vi "OAT Multistage Interpolation with IC.vi"(6 "initial state":cluster{"initial state":dbl[]}[](array[cluster]) {"initial state" format="%.2f"}, 8 "error in (no error)":errorcluster, 9 "filter":T1[](array[typedef]) {"coefficients" format="%.2f"}, 11 "X":dbl[](array[numeric]) format="%.2f") -> (0 "error out":errorcluster, 3 "Y":dbl[](array[numeric]) format="%.2f", 4 "final state":cluster{"final state":dbl[]}[](array[cluster]) {"final state" format="%.2f"})   [LabVIEW 2017, in "SoundVib_Resampling.lvlib"]
doc: "Interpolate the input sequence <B>X</B> with the multistage interpolation filter specified by <B>filter</B>."
uses:
  <vilib>/addons/Sound and Vibration/Order Analysis/Resample Order Tracking/SoundVib_Resampling.lvlib
  <vilib>/addons/_NISVFA/_Shared subVIs/Controls/OAT Decimation Filter.ctl
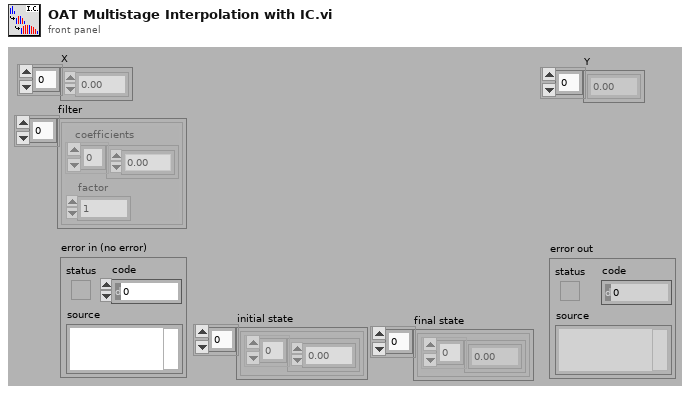
[diagram p1: front panel]
types:
  T1 = typedef "OAT Decimation Filter.ctl" = cluster{"coefficients":dbl[], "factor":i32}
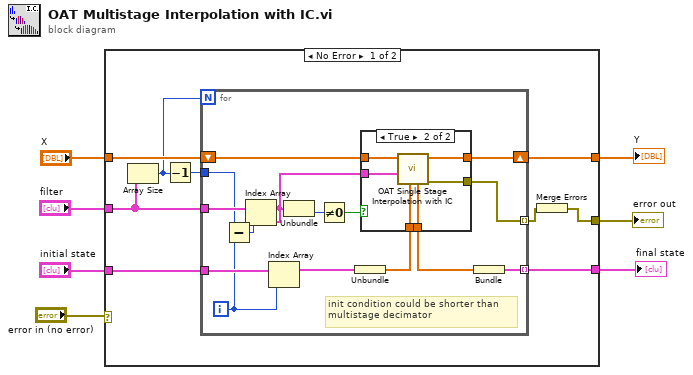
[diagram p0: block diagram]
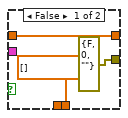
[diagram p2: hidden frame]
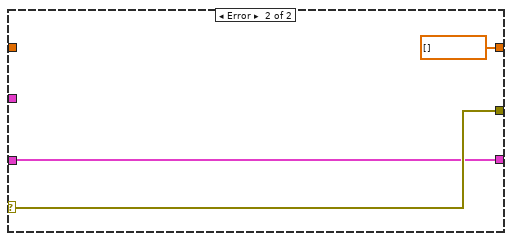
[diagram p3: hidden frame]
diagram:
  n1 = case shown="No Error" "error in (no error)" {
    selector: "error in (no error)" -> [_ w43]
    tunnel: "X" -> [w16 _]
    tunnel: [w15 w41] -> w6
    tunnel: [w14 dbl[] [] ("X")] -> w5
    tunnel: "initial state" -> [w13 w41]
    tunnel: "filter" -> [w12 _]
    tunnel: [w8 w43] -> w2
    frame No Error {
      n2 = Array Size(array=w12) -> (size(s)=w11:i32)
      n3 = Decrement(x=w11) -> (x-1=w10:i32)
      n4 = for {
        N: w11 -> [_]
        shift-right: [w27] -> w14
        shift-left: w16 -> [w29]
        tunnel: w12 -> [w28]
        tunnel: [w25] -> w15 mode=indexing
        tunnel: w13 -> [w23]
        tunnel: w10 -> [w18]
        tunnel: [w17] -> w9 mode=indexing
        i -> [w20]
        # "init condition could be shorter than \nmultistage decimator"
        n5 = Subtract(x=w18, y=w20) -> (x-y=w19:i32)
        n6 = Index Array(array=w28, index=w19) -> (element=w21:T1)
        n7 = Index Array(array=w23, index=w20) -> (element=w22:cluster{"initial state":dbl[]})
        n8 = Unbundle(w21) -> ("factor"=w31:i32)  [unwired: 1 out]
        n9 = Not Equal To 0?(x=w31) -> (x != 0?=w30:bool)
        n10 = Unbundle(w22) -> ("initial state"=w24:dbl[])
        n11 = case shown="True" w30 {
          tunnel: w29 -> [w34 w40]
          tunnel: w21 -> [_ w39]
          tunnel: [w34 w38] -> w27
          tunnel: [dbl[] [] ("final condition") w37] -> w26
          tunnel: w24 -> [_ w36]
          tunnel: [errorcluster {"status"=FALSE, "code"=0, "source"=""} ("error out") w35] -> w17
          frame False {
          }
          frame True {
            n12 = call <vilib>:"OAT Single Stage Interpolation with IC.vi"("initial state"=w36, "filter"=w39, "X"=w40) -> ("error out"=w35:errorcluster, "Y"=w38:dbl[], "final state"=w37:dbl[])  [unwired: 6 in]
          }
        }
        n13 = Bundle("final state"=w26) -> (w25:cluster{"final state":dbl[]})  [unwired: 1 in]
      }
      n14 = Merge Errors(w9) -> (w8:errorcluster)
    }
    frame Error {
    }
  }
  "Y" <- w5
  "final state" <- w6
  "error out" <- w2
